vi "Init Hardware.vi"(8 "error in (no error)":errorcluster, 11 "Red Pitaya Digitizer in":refnum<class "Red Pitaya Digitizer.lvclass">) -> (0 "error out":errorcluster, 3 "Red Pitaya Digitizer out":refnum<class "Red Pitaya Digitizer.lvclass">)   [LabVIEW 2024, in "Red Pitaya Digitizer.lvclass"]
uses:
  Red Pitaya Digitizer.lvclass
  Red Pitaya Digitizer.lvclass/Red Pitaya Digitizer.ctl
  RP Core/RP Instrument/RP Instrument.lvclass
  RP Command.ctl
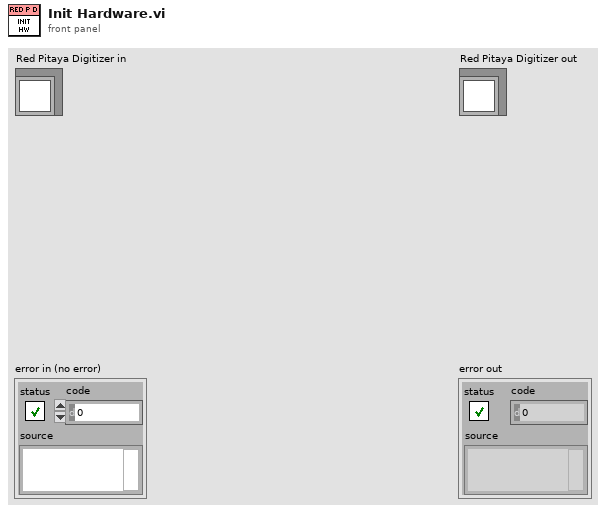
[diagram p1: front panel]
types:
  T1 = typedef "RP Command.ctl" = enum16{"Reset", "Read IDN", "Stop server", "Get status", "Get temperature", "Connect client", "Arm", "Software trigger", "Get whole buffer", "Get chunk", "System call", "Get config", "Set config", "Recieve data", "Recieve Calibartion", "Transmit data"}
  T2 = typedef "Pusle Driver Configuration.ctl" = cluster{"Post-trigger delay":dbl, "Post-trigger duration":dbl, "Rate":dbl, "Ranges":dbl[], "Re-name channels":string[], "Active channels":string, "External clock":bool}
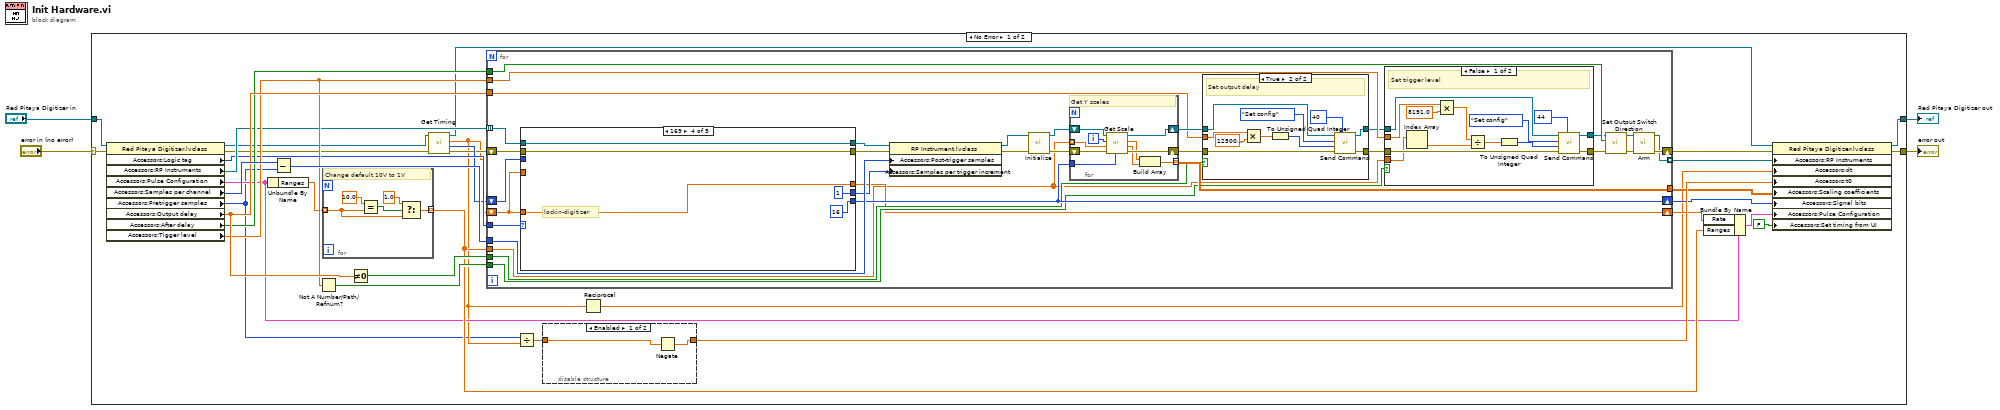
[diagram p0: block diagram]
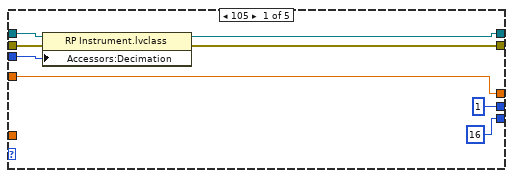
[diagram p5: hidden frame]
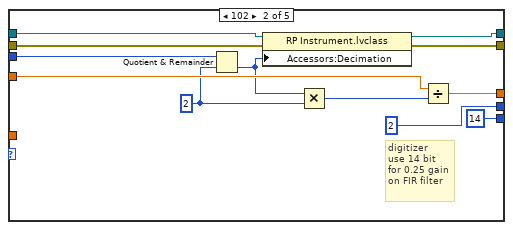
[diagram p6: hidden frame]
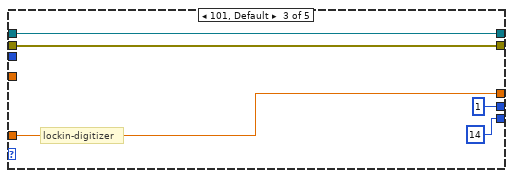
[diagram p7: hidden frame]
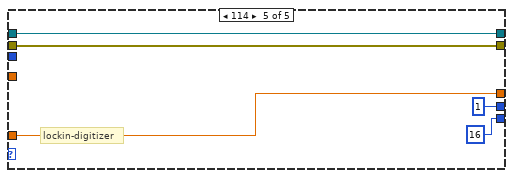
[diagram p8: hidden frame]
diagram:
  n1 = case shown="No Error" "error in (no error)" {
    selector: "error in (no error)" -> [w28 w150]
    tunnel: "Red Pitaya Digitizer in" -> [w37 w151]
    tunnel: [w33 w150] -> w2
    tunnel: [w32 w151] -> w1
    frame No Error {
      n2 = property class="Red Pitaya Digitizer.lvclass"(reference=w37, error in=w28) -> (reference out=w8:refnum<class "Red Pitaya Digitizer.lvclass">, error out=w11:errorcluster, "Accessors:Logic tag"=w14:u16, "Accessors:RP Instruments"=w21:refnum<class "RP Instrument.lvclass">[], "Accessors:Pulse Configuration"=w13:T2, "Accessors:Samples per channel"=w36:i32, "Accessors:Pretrigger samples"=w5:i32, "Accessors:Output delay"=w25:dbl, "Accessors:After delay"=w24:bool, "Accessors:Tigger level"=w22:dbl)
      n3 = Unbundle By Name(w13) -> ("Ranges"=w18:dbl[])
      n4 = Subtract(x=w36, y=w5) -> (x-y=w35:i32)
      n5 = Not A Number/Path/Refnum?(number/path/refnum=w22) -> (NaN/Path/Refnum?=w23:bool)
      n6 = for {
        tunnel: w18 -> [w147] mode=indexing
        tunnel: [w145] -> w17 mode=indexing
        # "Change default 10V to 1V"
        n7 = Equal?(x=10.0, y=w147) -> (x = y?=w148:bool)
        n8 = Select(t=1.0, s=w148, f=w147) -> (s? t:f=w145:dbl)
      }
      n9 = Not Equal To 0?(x=w25) -> (x != 0?=w26:bool)
      n10 = call-dynamic "Get Timing.vi"("error in (no error)"=w11, "Red Pitaya Digitizer in"=w8) -> ("error out"=w9:errorcluster, "Decimation"=w10:i32, "Rate"=w6:dbl, "Red Pitaya Digitizer out"=w7:refnum<class "Red Pitaya Digitizer.lvclass">)  [unwired: 6 in]
      n11 = for {
        tunnel: w35 -> [w71]
        tunnel: [w67] -> w29
        tunnel: w14 -> [w64]
        tunnel: w26 -> [w61]
        tunnel: w25 -> [w58]
        tunnel: w24 -> [w55]
        tunnel: w23 -> [w51]
        tunnel: w22 -> [w50]
        tunnel: w17 -> [w41]
        shift-right: [w69] -> w34
        shift-left: w9 -> [w48]
        shift-right: [w65] -> w27
        shift-left: w10 -> [w43]
        shift-right: [w44] -> w20
        shift-left: w6 -> [w42]
        tunnel: w21 -> [w47] mode=indexing
        tunnel: [w68] -> w16 mode=indexing
        n12 = case shown="169" w64 {
          tunnel: [16 ("Signal bits") 14 ("Signal bits") 14 ("Signal bits") 16 ("Signal bits") 16 ("Signal bits")] -> w65
          tunnel: [1 ("Samples per trigger increment") 2 ("Samples per trigger increment") 1 ("Samples per trigger increment") 1 ("Samples per trigger increment") 1 ("Samples per trigger increment")] -> w66
          tunnel: w43 -> [w105 w117 _ _ _]
          tunnel: w47 -> [w104 w116 w122 w127 w132]
          tunnel: [w103 w115 w122 w127 w132] -> w46
          tunnel: w48 -> [w102 w114 w121 w126 w131]
          tunnel: [w101 w113 w121 w126 w131] -> w45
          tunnel: w42 -> [_ _ w120 w125 w130]
          tunnel: [w100 w111 w120 w125 w130] -> w44
          tunnel: w42 -> [w100 w112 _ _ _]
          frame 105 {
            n13 = property class="RP Instrument.lvclass"(reference=w104, error in=w102, "Accessors:Decimation"=w105) -> (reference out=w103:refnum<class "RP Instrument.lvclass">, error out=w101:errorcluster)
          }
          frame 102 {
            w110 = 2 ("y")
            # "digitizer\nuse 14 bit \nfor 0.25 gain\non FIR filter"
            n14 = Quotient & Remainder(x=w117, y=w110) -> (floor(x/y)=w109:i32)  [unwired: 1 out]
            n15 = property class="RP Instrument.lvclass"(reference=w116, error in=w114, "Accessors:Decimation"=w109) -> (reference out=w115:refnum<class "RP Instrument.lvclass">, error out=w113:errorcluster)
            n16 = Multiply(x=w109, y=w110) -> (x*y=w108:i32)
            n17 = Divide(x=w112, y=w108) -> (x/y=w111:dbl)
          }
          frame 101, Default {
            # "lockin-digitizer"
          }
          frame 169 {
            # "lockin-digitizer"
          }
          frame 114 {
            # "lockin-digitizer"
          }
        }
        n18 = property class="RP Instrument.lvclass"(reference=w46, error in=w45, "Accessors:Post-trigger samples"=w71, "Accessors:Samples per trigger increment "=w66) -> (reference out=w72:refnum<class "RP Instrument.lvclass">, error out=w70:errorcluster)
        n19 = call-dynamic "Initialize.vi"("error in (no error)"=w70, "RP Instrument in"=w72) -> ("error out"=w62:errorcluster, "RP Instrument out"=w63:refnum<class "RP Instrument.lvclass">)  [unwired: 8 in]
        n20 = for {
          tunnel: w41 -> [w136] mode=indexing
          tunnel: [w144] -> w67 mode=indexing
          tunnel: w65 -> [w135]
          shift-right: [w142] -> w59
          shift-left: w63 -> [w143]
          shift-right: [w140] -> w60
          shift-left: w62 -> [w141]
          i -> [w137]
          # "Get Y scales"
          n21 = call-dynamic "Get Scale.vi"("Signal bits"=w135, "error in (no error)"=w141, "Range"=w136, "Channel"=w137, "RP Instrument in"=w143) -> ("error out"=w140:errorcluster, "slope"=w138:dbl, "y intersept"=w139:dbl, "RP Instrument out"=w142:refnum<class "RP Instrument.lvclass">)  [unwired: 2 in, 1 out]
          n22 = Build Array(w139, w138) -> (w144:dbl[])
        }
        n23 = case shown="True" w61 {
          tunnel: w60 -> [w88 w94]
          tunnel: w59 -> [w89 w93]
          tunnel: w58 -> [_ w92]
          tunnel: [w88 w91] -> w54
          tunnel: [w89 w90] -> w49
          frame False {
          }
          frame True {
            # "Set output delay"
            n24 = Multiply(x=w92, y=125000000.0) -> (x*y=w98:dbl)
            n25 = To Unsigned Quad Integer(1:w98) -> (0:w99:u64)
            n26 = call-dynamic "Send Command.vi"("Config offset"=u64 40, "error in (no error)"=w94, "Command payload"=w99, "Command number"=RP_Command."Set config", "RP Instrument in"=w93) -> ("error out"=w91:errorcluster, "RP Instrument out"=w90:refnum<class "RP Instrument.lvclass">)  [unwired: 5 in]
          }
        }
        n27 = case shown="False" w51 {
          tunnel: w54 -> [w81 w86]
          tunnel: w49 -> [w77 w87]
          tunnel: w50 -> [w80 _]
          tunnel: [w79 w86] -> w53
          tunnel: [w78 w87] -> w52
          tunnel: w41 -> [w76 _]
          frame False {
            # "Set trigger level"
            n28 = Index Array(array=w76) -> (element=w73:dbl)  [unwired: 1 in]
            n29 = Multiply(x=w80, y=8191.0) -> (x*y=w74:dbl)
            n30 = Divide(x=w74, y=w73) -> (x/y=w75:dbl)
            n31 = To Unsigned Quad Integer(1:w75) -> (0:w85:u64)
            n32 = call-dynamic "Send Command.vi"("Config offset"=u64 44, "error in (no error)"=w81, "Command payload"=w85, "Command number"=RP_Command."Set config", "RP Instrument in"=w77) -> ("error out"=w79:errorcluster, "RP Instrument out"=w78:refnum<class "RP Instrument.lvclass">)  [unwired: 5 in]
          }
          frame True {
          }
        }
        n33 = call-dynamic "Set Output Switch Direction.vi"("error in (no error)"=w53, "After delay"=w55, "RP Instrument in"=w52) -> ("error out"=w57:errorcluster, "RP Instrument out"=w56:refnum<class "RP Instrument.lvclass">)  [unwired: 7 in]
        n34 = call-dynamic "Arm.vi"("error in (no error)"=w57, "RP Instrument in"=w56) -> ("error out"=w69:errorcluster, "RP Instrument out"=w68:refnum<class "RP Instrument.lvclass">)  [unwired: 8 in]
      }
      n35 = Divide(x=w5, y=w6) -> (x/y=w31:dbl)
      n36 = disable-structure shown="Enabled" {
        disable-tunnel: w31 -> [w39 w40]
        disable-tunnel: [w38 w40] -> w30
        frame Enabled {
          n37 = Negate(x=w39) -> (-x=w38:dbl)
        }
        frame Disabled {
        }
      }
      n38 = Reciprocal(x=w6) -> (1/x=w12:dbl)
      n39 = Bundle By Name(cluster=w13, "Rate"=w20, "Ranges"=w17) -> (w19:T2)
      n40 = property class="Red Pitaya Digitizer.lvclass"(reference=w7, error in=w34, "Accessors:RP Instruments"=w16, "Accessors:dt"=w12, "Accessors:t0"=w30, "Accessors:Scaling coefficients"=w29, "Accessors:Signal bits"=w27, "Accessors:Pulse Configuration"=w19, "Accessors:Set timing from UI"=FALSE ("Set timing from UI")) -> (reference out=w32:refnum<class "Red Pitaya Digitizer.lvclass">, error out=w33:errorcluster)
    }
    frame Error {
    }
  }
  "error out" <- w2
  "Red Pitaya Digitizer out" <- w1
